vi "nanocal-frontend-client-standalone-18.vi"() -> ()   [LabVIEW 2018]
uses:
  frontend -- data type -- folder/frontend -- data type.ctl
  nanocal/Nanocalorimetry/data/NanoCalLib.lvlibp
panel:
  out "Ts (K)":dbl
  out "output cluster 2":T1
  in  "wait (ms)":u32=100
  in  "Stop":bool
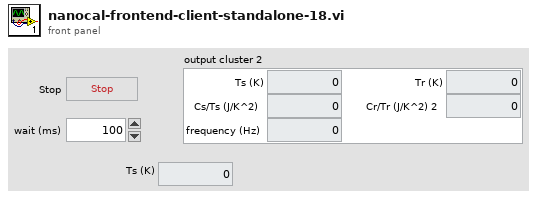
[diagram p1: front panel]
types:
  T1 = typedef "frontend -- data type.ctl" = cluster{"frequency (Hz)":dbl, "Cs/Ts (J/K^2)":dbl, "Ts (K)":dbl, "Cr/Tr (J/K^2) 2":dbl, "Tr (K)":dbl}
  T2 = typedef "NanoCalLib.lvlibp/NanoReadings.lvlib/NanoReadings_Parameters_TypeDef.ctl" = cluster{"Power":T3, "C and K":T4, "IV dc":T5, "Tdc,Tac":T6, "Phases":T7, "f etc":T8, "IV 1st harm":T9, "ForAveraging":cluster{"SinTherm":dbl[], "CosTherm":dbl[], "SinHeats":dbl[], "CosHeats":dbl[]}, "Output":T10, "Magnetic field etc.":T11, "Calibration":T12, "CT etc":T13, "IV 2nd harm":T14, "Resistance":T15, "Time etc":T16}
  T3 = typedef "NanoCalLib.lvlibp/NanoReadings.lvlib/NanoReadings_Power.ctl" = cluster{"PHs (W)":dbl, "PHr (W)":dbl, "Ps,dc (W)":dbl, "Pr,dc (W)":dbl, "PHs,dc (W)":dbl, "PHr,dc (W)":dbl, "Ps,ac (W)":dbl, "Pr,ac (W)":dbl, "PHs/PHr":dbl, "Poffs (W)":dbl, "Ps total (W)":dbl, "Pr total (W)":dbl, "Ps-Pr total (W)":dbl, "Ps,offs (W)":dbl}
  T4 = typedef "NanoCalLib.lvlibp/NanoReadings.lvlib/NanoReadings_CandK.ctl" = cluster{"Cs (J/K)":dbl, "Ks (W/K)":dbl, "Cr (J/K)":dbl, "Kr (W/K)":dbl, "Cdiff (J/K)":dbl, "Cs-Cr (J/K)":dbl, "Cdiff old style (J/K)":dbl, "Cr from S,diff (J/K)":dbl}
  T5 = typedef "NanoCalLib.lvlibp/NanoReadings.lvlib/NanoReadings_IandV.ctl" = cluster{"Is,dc (A)":dbl, "Ir,dc (A)":dbl, "Us,dc (V)":dbl, "Ur,dc (V)":dbl, "Udiff,dc (V)":dbl, "IHs dc (A)":dbl, "UHs dc (V)":dbl, "IHr dc (A)":dbl, "UHr dc (V)":dbl, "Uoffs dc (V)":dbl, "Ioffs dc (A)":dbl}
  T6 = typedef "NanoCalLib.lvlibp/NanoReadings.lvlib/NanoReadings_TdcTac.ctl" = cluster{"Ts (K)":dbl, "Tr (K)":dbl, "Tdiff from Rs,Rr":dbl, "Tdiff from Udiff (K)":dbl, "Ts,ac (K)":dbl, "Tr,ac (K)":dbl, "Tdiff,ac (K)":dbl, "Ts,ac driftcorr (K)":dbl, "Tr,ac driftcorr (K)":dbl, "Tr,ac from Ts,diff,ac (K)":dbl, "T target (K)":dbl}
  T7 = typedef "NanoCalLib.lvlibp/NanoReadings.lvlib/NanoReadings_Phases.ctl" = cluster{"Phi Is (deg)":dbl, "Phi Us (deg)":dbl, "Phi Ir (deg)":dbl, "Phi Ur (deg)":dbl, "Phi Udiff (deg)":dbl, "Phi IHs (deg)":dbl, "Phi UHs (deg)":dbl, "Phi IHr (deg)":dbl, "Phi UHr (deg)":dbl, "Phi R from S,diff (deg)":dbl, "Phi Is 1st (deg)":dbl, "Phi Us 1st (deg)":dbl, "Phi Ir 1st (deg)":dbl, "Phi Ur 1st (deg)":dbl, "Phi Udiff 1st (deg)":dbl, "Phi Udiff, raw (deg)":dbl}
  T8 = typedef "NanoCalLib.lvlibp/NanoReadings.lvlib/NanoReadings_Frequencies.ctl" = cluster{"f (Hz)":dbl, "f therm (Hz)":dbl, "omega (rad/s)":dbl, "Tan Phi S/diff":dbl, "Sin Phi":dbl, "Cos Phi":dbl, "f mix (Hz)":dbl, "tau (s)":dbl}
  T9 = typedef "NanoCalLib.lvlibp/NanoReadings.lvlib/NanoReadings_FirstHarmonic.ctl" = cluster{"Is,ac 1st (A)":dbl, "Ir,ac 1st (A)":dbl, "Us,ac 1st (V)":dbl, "Ur,ac 1st (V)":dbl, "Udiff,ac 1st (V)":dbl, "IHs (A)":dbl, "UHs (V)":dbl, "IHr (A)":dbl, "UHr (V)":dbl}
  T10 = typedef "NanoCalLib.lvlibp/NanoReadings.lvlib/NanoReadings_Output.ctl" = cluster{"S phase (deg)":dbl, "R phase (deg)":dbl, "Hs ac out (Vrms)":dbl, "Hr ac out (Vrms)":dbl, "S Therm dc out (V)":dbl, "R Therm dc out (V)":dbl, "S Therm ac out (Vrms)":dbl, "R Therm ac out (Vrms)":dbl, "Offset dc out (V)":dbl, "Hs dc out (V)":dbl, "Hr dc out (V)":dbl, "Offset ac out (Vrms)":dbl}
  T11 = typedef "NanoCalLib.lvlibp/NanoReadings.lvlib/NanoReadings_MagneticFieldEtc.ctl" = cluster{"H (T)":dbl, "T probe (K)":dbl, "Polar angle (deg)":dbl, "Azimuthal angle (deg)":dbl}
  T12 = typedef "NanoCalLib.lvlibp/NanoReadings.lvlib/NanoReadings_Calibration.ctl" = cluster{"1+Rs/RIs factor":dbl, "1+RIs/Rs factor":dbl, "Rs,scaled (ohm)":dbl, "Rr,scaled (ohm)":dbl, "R lead S (ohm)":dbl, "R lead R (ohm)":dbl, "|dlnR/dlnT| S":dbl, "|dlnR/dlnT| R":dbl, "dTs/dt (mK/s)":dbl, "dTr/dt (mK/s)":dbl}
  T13 = typedef "NanoCalLib.lvlibp/NanoReadings.lvlib/NanoReadings_CTetc.ctl" = cluster{"Cs/T (J/K^2)":dbl, "Cr/T (J/K^2)":dbl, "Cdiff/T (J/K^2)":dbl, "(Cs-Cr)/T (J/K^2)":dbl, "Cdiff/T old style (J/K^2)":dbl, "Cr/T from S,diff (J/K^2)":dbl, "Ts^2 (K^2)":dbl, "Tr^2 (K^2)":dbl}
  T14 = typedef "NanoCalLib.lvlibp/NanoReadings.lvlib/NanoReadings_2ndHarmonic.ctl" = cluster{"Is,ac (A)":dbl, "Ir,ac (A)":dbl, "Us,ac (V)":dbl, "Ur,ac (V)":dbl, "Udiff,ac (V)":dbl}
  T15 = typedef "NanoCalLib.lvlibp/NanoReadings.lvlib/NanoReadings_Resistance.ctl" = cluster{"RHs (ohm)":dbl, "RHr (ohm)":dbl, "Rs (ohm)":dbl, "Rr (ohm)":dbl, "RHs,dc (ohm)":dbl, "RHr,dc (ohm)":dbl, "Rs,ac (ohm)":dbl, "Rr,ac (ohm)":dbl, "Roffs (ohm)":dbl}
  T16 = typedef "NanoCalLib.lvlibp/NanoReadings.lvlib/NanoReadings_TimeEtc.ctl" = cluster{"Time (s)":dbl, "Datapoint index":dbl, "Datapoint time (s)":dbl}
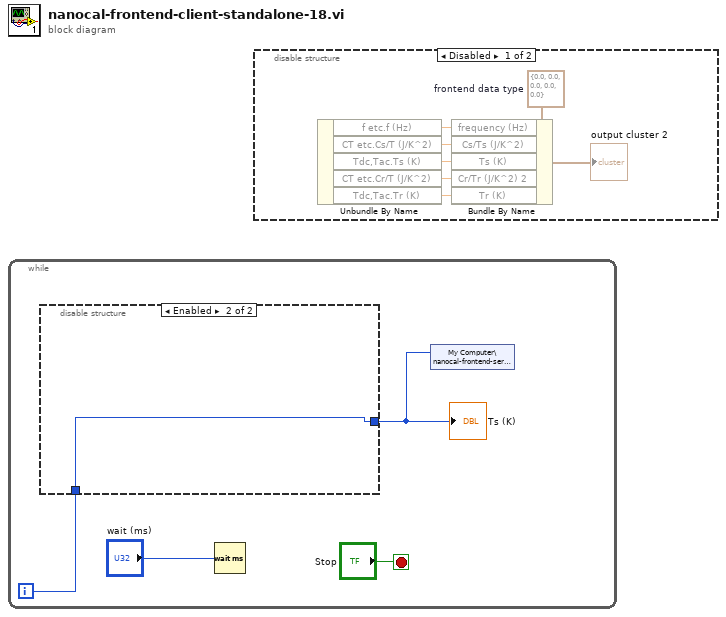
[diagram p0: block diagram]
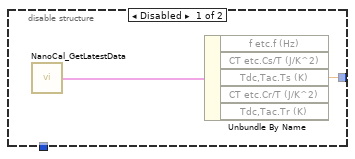
[diagram p3: hidden frame]
diagram:
  n1 = while {
    i -> [w1]
    stop <- "Stop" stop-if-true
    n2 = disable-structure shown="Enabled" {
      disable-tunnel: [w6 w7] -> w2
      disable-tunnel: w1 -> [_ w7]
      frame Disabled {
        n3 = call "NanoCal_GetLatestData.vi"() -> ("Latest data"=w5:T2)  [unwired: 1 in]
        n4 = Unbundle By Name(w5) -> ("Tdc,Tac.Ts (K)"=w6:dbl)  [unwired: 4 out]
      }
      frame Enabled {
      }
    }
    "Ts (K)" <- w2
    n5 = Wait (ms)(milliseconds to wait="wait (ms)") -> ()  [unwired: 1 out]
    n6 = shared-variable "My Computer\\nanocal-frontend-server-data-LV18.lvlib\\data-Ts"(w2) -> ()  [unwired: 1 in, 1 out]
  }
  n7 = disable-structure shown="Disabled" {
    frame Disabled {
      w14 = T1 {"frequency (Hz)"=0.0, "Cs/Ts (J/K^2)"=0.0, "Ts (K)"=0.0, "Cr/Tr (J/K^2) 2"=0.0, "Tr (K)"=0.0}  # frontend data type
      n8 = Unbundle By Name() -> ("f etc.f (Hz)"=w11:dbl, "CT etc.Cs/T (J/K^2)"=w13:dbl, "Tdc,Tac.Ts (K)"=w12:dbl, "CT etc.Cr/T (J/K^2)"=w10:dbl, "Tdc,Tac.Tr (K)"=w9:dbl)  [unwired: 1 in]
      n9 = Bundle By Name(cluster=w14, "frequency (Hz)"=w11, "Cs/Ts (J/K^2)"=w13, "Ts (K)"=w12, "Cr/Tr (J/K^2) 2"=w10, "Tr (K)"=w9) -> (→"output cluster 2":T1)
    }
    frame Enabled {
    }
  }
